vi "SVFA Zoom Power Spectral Density (1 Ch).vi"(0 "scaled signal [EU]":waveform(dbl)={"t0"=timestamp(0 s since 1904-01-01), "dt"=0.0001, "Y"=[]}, 3 "zoom settings":T2={"frequency range"={"start frequency"=1000.0, "stop frequency"=2000.0}, "window"=1, "number of lines"=400, "% overlap"=0.0} {"% overlap" min=0.0 format="%.2f"; "number of lines" min=2; "window" items=["None ", "Hanning", "Hamming", "Blackman-Harris", "Exact Blackman", "Blackman", "Flat Top", "4 Term B-Harris ", "7 Term B-Harris", "Low Sidelobe"]; "frequency range"."stop frequency" min=0.0 format="%.2f"; "frequency range"."start frequency" min=0.0 format="%.2f"}, 4 "dB On (F)":bool, 5 "error in (no error)":errorcluster, 6 "desired units":enum16{"EU^2 / Hz", "EU / sqrt(Hz)"}(ring), 7 "averaging parameters":T1={"averaging mode"=enum."No averaging", "weighting mode"=enum."Exponential", "number of averages"=10, "linear mode"=enum."One shot"} {"number of averages" min=1 step=1}, 9 "restart averaging (F)":bool) -> (11 "averaging done":bool, 12 "new spectrum available":bool, 13 "averages completed":dbl, 14 "power spectral density [EU^2 rms / Hz]":cluster{"f0":dbl, "df":dbl, "magnitude":dbl[]}={"f0"=nan, "df"=inf, "magnitude"=[]} {"magnitude" format="%.2p"; "df" format="%.2p"; "f0" format="%.2p"}, 15 "unit label":string, 18 "spectrum info":T3={"channel name"="", "description"="", "x-axis units"=1, "spectral info"={"spectrum type"=enum."Power [Magnitude^2]", "linear/dB"=enum."linear", "window"=0, "window size"=0, "FFT size"=0}, "engineering units"=0, "custom label"="", "dB reference [EU]"=0.0, "peak units"=enum."rms", "weighting filter"=0, "spectral density?"=FALSE, "unit label"="", "spectrum skewed?"=FALSE, "complimentary spectrum units"=enum."none"} {"x-axis units" items=["Time (s)"=0, "Frequency-CB (Hz)"=1, "Frequency-CPB (Hz)"=1248, "Frequency-Arbitrary (Hz)"=2357, "Quefrency (s)"=2, "Revolutions (rev)"=3, "Order"=4, "Speed (RPM)"=11, "Speed (rad/s)"=21, "Index"=65535]; "weighting filter" items=["Linear", "A-weighting", "B-weighting", "C-weighting", "ITU-R 468-4", "Dolby", "CCITT", "C-message", "Wb", "Wc", "Wd", "We", "Wf", "Wh", "Wj", "Wk", "Wm", "AES17 20 kHz lowpass", "AES17 40 kHz lowpass", "AES17 20 kHz highpass", "AES17 40 kHz highpass"]; "dB reference [EU]" format="%.2f"; "engineering units" items=["custom..."=0, "V"=1, "A"=21, "C"=30, "pC"=31, "s"=32, "-"=29, "Pa"=2, "N"=20, "g"=3, "m/s^2"=4, "m/s"=5, "m"=6, "mm/s"=12, "mm"=13, "micron/s"=14, "micron"=15, "in/s^2"=7, "in/s"=8, "in"=9, "mil/s"=10, "mil"=11, "rad/s^2"=16, "rad/s"=17, "rad"=18, "deg/s^2"=26, "deg/s"=27, "deg"=28, "RPM"=22, "cycle/s^2"=23, "Hz"=24, "cycle"=25, "strain"=19]; "spectral info"."window" items=["None "=0, "Hanning"=1, "Hamming"=2, "Blackman-Harris"=3, "Exact Blackman"=4, "Blackman"=5, "Flat Top"=6, "4 Term B-Harris "=7, "7 Term B-Harris"=8, "Low Sidelobe"=9, "Force - Exponential"=10, "Gaussian"=62]}, 19 "error out":errorcluster)   [LabVIEW 2017]
doc: "Computes the zoom power spectral density of <B>scaled signal [EU]</B> and <B>zoom settings</B>. Data accumulates each time this VI is called. However, it returns a new spectrum only when sufficient data accumulates. Indicators and subsequent processing should only be called when <B>new spectrum available</B> is TRUE. Wire data to the <B>scaled signal [EU]</B> input to determine the polymorphic instance to use or manually select the instance."
uses:
  <vilib>/addons/_NISVFA/_Shared subVIs/Controls/svc_Spectrum Info.ctl
  <vilib>/addons/_NISVFA/_Shared subVIs/Controls/svc_X-Axis Units.ctl
  <vilib>/addons/_NISVFA/_Shared subVIs/Controls/svc_Spectrum Type.ctl
  <vilib>/addons/_NISVFA/_Shared subVIs/Controls/svc_Engineering Units Text Ring.ctl
  <vilib>/addons/_NISVFA/_Shared subVIs/Controls/svc_Weighting Filter Text Ring.ctl
  <vilib>/addons/_NISVFA/_Shared subVIs/Controls/svc_Complimentary Spectrum Units.ctl
  <vilib>/addons/_NISVFA/_Spectrum Processing/SVFA Unit Conversion (1 Ch).vi
  <vilib>/addons/_NISVFA/_Shared subVIs/Common/svc_Get SV Channel Info.vi
  <vilib>/addons/_NISVFA/_Shared subVIs/Common/svc_Spectrum Units.vi
  <vilib>/addons/_NISVFA/_Shared subVIs/Spectrum Averaging/svfa_Reset Averaging State Info.vi
  <vilib>/addons/_NISVFA/_Shared subVIs/Spectrum Averaging/svfa_Average Array with Avg Checks (complex) No State.vi
  <vilib>/addons/_NISVFA/_Shared subVIs/Common/svc_Complex to Mag2 Array.vi
  <vilib>/addons/_NISVFA/_Shared subVIs/Spectrum Averaging/svfa_Average Array with Avg Checks (real) No State.vi
  <vilib>/addons/_NISVFA/_Spectrum Processing/subVIs/svfa_Conversion Utility (spectrum info).vi
  <vilib>/addons/_NISVFA/_Shared subVIs/Spectrum Averaging/svfa_Average Array (complex) No State.vi
  <vilib>/addons/_NISVFA/_Shared subVIs/Spectrum Averaging/svfa_Average Array (real) No State.vi
  <vilib>/addons/_NISVFA/_Spectrum Processing/subVIs/svfa_Peak to RMS to Peak2Peak.vi
  <vilib>/addons/_NISVFA/_Spectrum Processing/subVIs/svfa_Mag to Mag2.vi
  <vilib>/addons/_NISVFA/_Spectrum Processing/subVIs/svfa_Linear to dB.vi
  <vilib>/addons/_NISVFA/_Spectrum Processing/subVIs/svfa_dBrefA to dBrefB.vi
  <vilib>/addons/_NISVFA/_Spectrum Processing/subVIs/svfa_Spectrum to Spectral Density.vi
  <vilib>/addons/_NISVFA/_Shared subVIs/Spectrum Averaging/svfa_No Average Array (complex).vi
  <vilib>/addons/_NISVFA/_Shared subVIs/Spectrum Averaging/svfa_Average Array (complex).vi
  <vilib>/addons/_NISVFA/_Shared subVIs/Spectrum Averaging/svfa_No Average Array (real).vi
  <vilib>/addons/_NISVFA/_Shared subVIs/Spectrum Averaging/svfa_Average Array (real).vi
  <vilib>/addons/_NISVFA/_Shared subVIs/Spectrum Averaging/svfa_Peak Hold Array.vi
  <vilib>/addons/_NISVFA/_Shared subVIs/Common/svc_Get Weighting Enum and Labels.vi
  <vilib>/addons/_NISVFA/_Shared subVIs/Common/svc_Unit Label Lexical Class.vi
  <vilib>/addons/_NISVFA/_Shared subVIs/Common/svc_Engineering Units to Unit Label.vi
  <vilib>/addons/_NISVFA/_Shared subVIs/Common/svc_Format Value (DBL).vi
  <vilib>/addons/_NISVFA/_Shared subVIs/Common/svc_Window Parameters.vi
  <vilib>/addons/_NISVFA/_Shared subVIs/Common/svc_Channel Info to Spectrum Info.vi
  <vilib>/addons/_NISVFA/_Shared subVIs/Common/svc_Unit Label to Engineering Units.vi
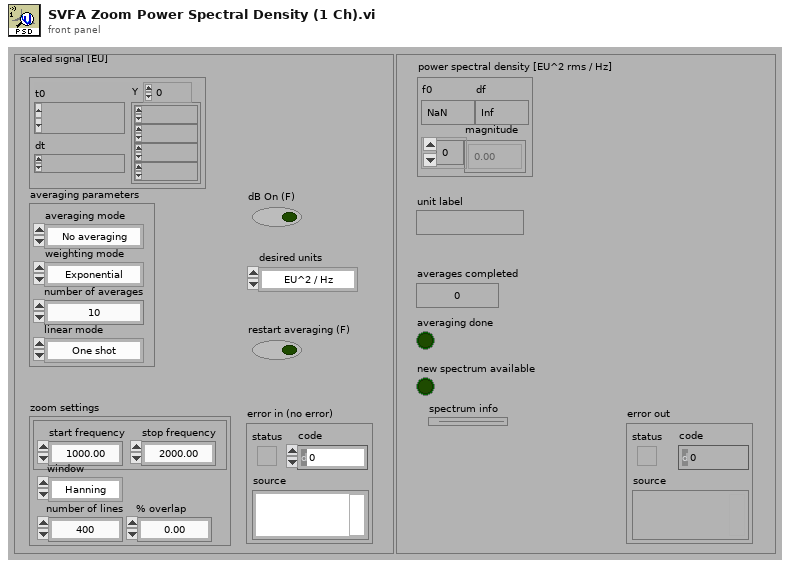
[diagram p1: front panel]
types:
  T1 = cluster{"averaging mode":enum16{"No averaging", "Vector averaging", "RMS averaging", "Peak hold"}, "weighting mode":enum16{"Linear", "Exponential"}, "number of averages":u32, "linear mode":enum16{"One shot", "Auto restart"}}
  T2 = cluster{"frequency range":cluster{"start frequency":dbl, "stop frequency":dbl}, "window":u16, "number of lines":i32, "% overlap":dbl}
  T3 = typedef "svc_Spectrum Info.ctl" = cluster{"channel name":string, "description":string, "x-axis units":T4, "spectral info":cluster{"spectrum type":T5, "linear/dB":enum16{"linear", "dB"}, "window":u16, "window size":i32, "FFT size":i32}, "engineering units":T6, "custom label":string, "dB reference [EU]":dbl, "peak units":enum16{"rms", "peak", "peak-peak"}, "weighting filter":T7, "spectral density?":bool, "unit label":string, "spectrum skewed?":bool, "complimentary spectrum units":T8}
  T4 = typedef "svc_X-Axis Units.ctl" = u16
  T5 = typedef "svc_Spectrum Type.ctl" = enum16{"FFT Spectrum [complex]", "Amplitude [Magnitude]", "Power [Magnitude^2]", "Cross Spectrum [complex]", "Frequency Response [Complex]"}
  T6 = typedef "svc_Engineering Units Text Ring.ctl" = u16
  T7 = typedef "svc_Weighting Filter Text Ring.ctl" = u16
  T8 = typedef "svc_Complimentary Spectrum Units.ctl" = enum16{"none", "radians", "degrees", "cycles", "imaginary"}
  T9 = enum16{"Restart processing", "Continue processing", "Skip processing"}
  T10 = enum16{"No averaging", "Vector averaging", "RMS averaging", "Peak hold"}
  T11 = cluster{"linear/dB":enum16{"no change", "linear", "dB"}, "dB reference (0: no change)":dbl, "power/magnitude":enum16{"no change", "power", "magnitude"}, "view":enum16{"no change", "rms", "peak", "peak-peak"}}
  T12 = enum16{"no change", "spectrum", "spectral density"}
  T13 = cluster{"zoom settings":cluster{"center frequency":dbl, "zoom":i32, "trim":dbl}, "FFT settings":cluster{"window":enum16{"None ", "Hanning", "Hamming", "Blackman-Harris", "Exact Blackman", "Blackman", "Flat Top", "4 Term B-Harris ", "7 Term B-Harris", "Low Sidelobe"}, "window size":i32, "FFT size":i32, "%overlap":dbl}}
  T14 = cluster{"complex FFT":cdb[], "real FFT":dbl[], "f0":dbl, "df":dbl, "averages completed":dbl, "averaging parameters":cluster{"averaging mode":enum16{"No averaging", "Vector averaging", "RMS averaging", "Peak hold"}, "weighting mode":enum16{"Linear", "Exponential"}, "number of averages":u32, "linear mode":enum16{"One shot", "Auto restart"}}}
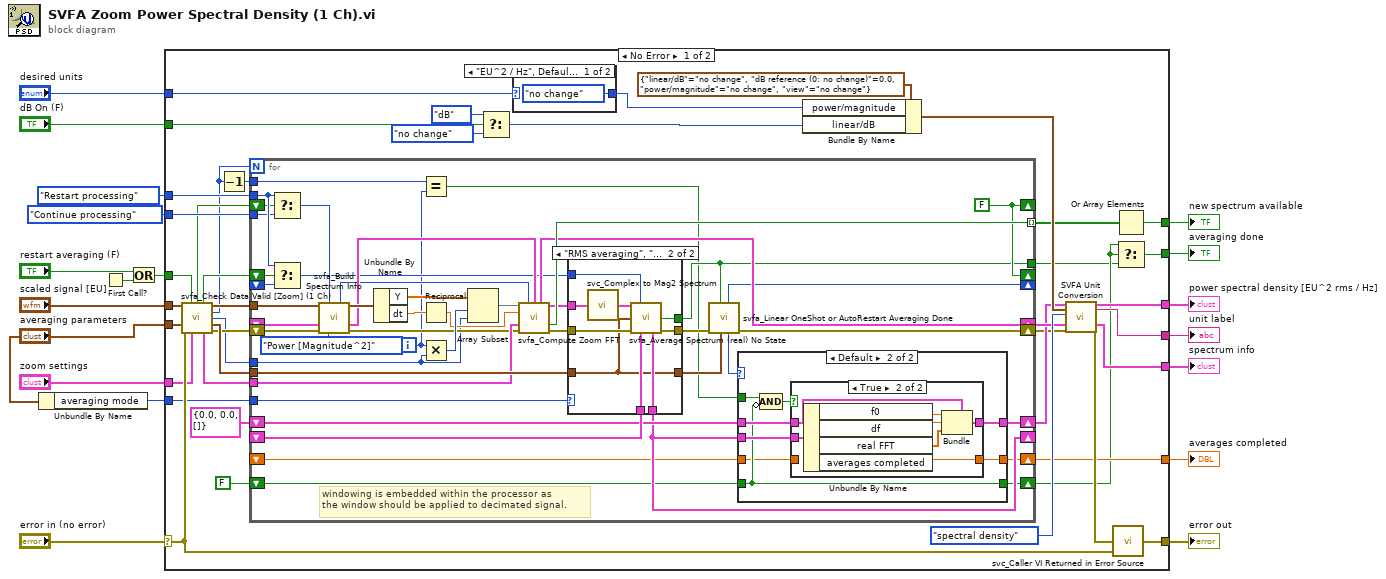
[diagram p0: block diagram]
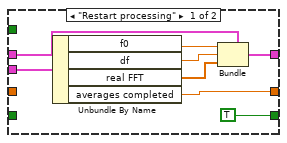
[diagram p2: hidden frame]
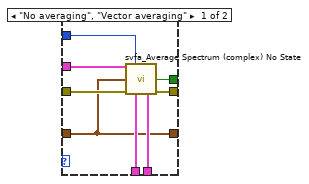
[diagram p4: hidden frame]
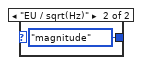
[diagram p5: hidden frame]
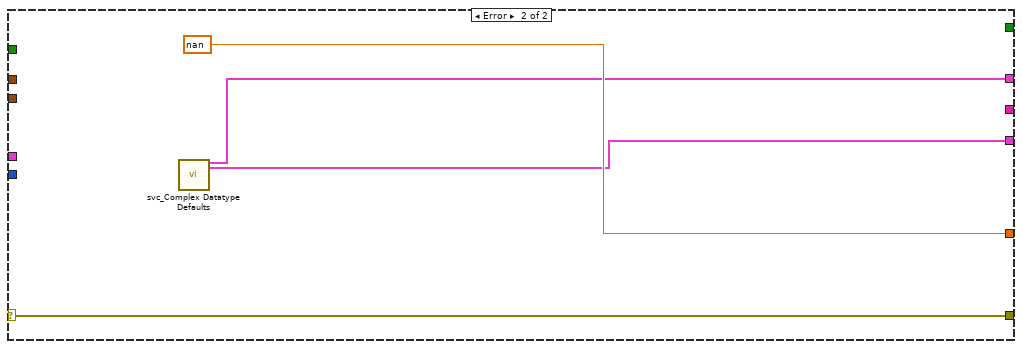
[diagram p6: hidden frame]
diagram:
  n1 = Unbundle By Name("averaging parameters") -> ("averaging mode"=w1:T10)
  n2 = First Call?() -> (First Call?: T/F=w8:bool)
  n3 = Or(x="restart averaging (F)", y=w8) -> (x .or. y?=w6:bool)
  n4 = case shown="No Error" "error in (no error)" {
    tunnel: [w24 nan ("Averaged So-far")] -> w18
    tunnel: [w60 w152] -> w14
    tunnel: "averaging parameters" -> [w56 _]
    tunnel: "zoom settings" -> [w41 _]
    tunnel: "scaled signal [EU]" -> [w61 _]
    tunnel: [w58 _] -> w13
    tunnel: "dB On (F)" -> [w47 _]
    tunnel: [w57 w151] -> w12
    tunnel: w6 -> [w34 _]
    tunnel: "desired units" -> [w48 _]
    selector: "error in (no error)" -> [w54 w154]
    tunnel: [w55 w154] -> w16
    tunnel: [w35 _] -> w17
    tunnel: [w22 _] -> w10
    tunnel: T9."Restart processing" ("processing control") -> [w33 _]
    tunnel: T9."Continue processing" ("processing control") -> [w32 _]
    tunnel: w1 -> [w30 _]
    frame No Error {
      n5 = call <vilib>:"svfa_Check Data Valid [Zoom] (1 Ch).vi"("signal [V]"=w61, "restart averaging (F)"=w34, "averaging parameters"=w56, "error in (no error)"=w54, "zoom settings"=w41) -> ("reset processing"=w31:bool, "restart averaging"=w39:bool, "dup signal [V]"=w44:waveform(dbl), "iterations"=w29:i32, "maximum block size"=w36:i32, "dup averaging parameters"=w43:T1, "zoom FFT settings"=w40:T13, "error out"=w42:errorcluster)  [unwired: 3 in]
      n6 = Decrement(x=w29) -> (x-1=w28:i32)
      n7 = for {
        N: w29 -> [_]
        tunnel: [w105] -> w38 mode=indexing
        tunnel: w44 -> [w106]
        tunnel: [w74] -> w21
        shift-left: _ -> [w102]
        shift-right: [w70] -> _
        shift-right: [w104] -> w37
        shift-left: _ -> [w103]
        tunnel: w43 -> [w101]
        shift-right: [w73] -> _
        shift-left: _ -> [w99]
        tunnel: w33 -> [w95]
        tunnel: w40 -> [w97]
        shift-right: [w76] -> _
        shift-left: w39 -> [w98]
        tunnel: w36 -> [w75]
        tunnel: w32 -> [w94]
        shift-right: [w76] -> _
        shift-left: w31 -> [w93]
        tunnel: w30 -> [w78]
        shift-right: [w72] -> w25
        shift-left: cluster{"f0":dbl, "df":dbl, "real FFT":dbl[]} {"f0"=0.0, "df"=0.0, "real FFT"=[]} -> [w71]
        tunnel: w28 -> [w69]
        shift-right: [w65] -> w24
        shift-left: _ -> [w64]
        shift-right: [w66] -> w23
        shift-left: FALSE ("restart averaging") -> [w63]
        shift-right: [w62] -> w20
        shift-left: w42 -> [w100]
        i -> [w68]
        w76 = FALSE ("restart averaging")
        # "windowing is embedded within the processor as \nthe window should be applied to decimated signal."
        n8 = Select(t=w95, s=w93, f=w94) -> (s? t:f=w80:T9)
        n9 = Select(t=w95, s=w98, f=w99) -> (s? t:f=w79:T9)
        n10 = call <vilib>:"svfa_Build Spectrum Info.vi"("scaled signal [EU]"=w106, "processing control"=w80, "spectrum info in"=w103, "error in (no error)"=w100, "spectrum type"=svc_Spectrum_Type."Power [Magnitude^2]") -> ("dup processing control"=w85:T9, "dup scaled signal [EU]"=w91:waveform(dbl), "spectrum info out"=w89:T3, "error out"=w83:errorcluster)  [unwired: 7 in]
        n11 = Unbundle By Name ("Get Waveform Components")(w91) -> ("Y"=w82:dbl[], "dt"=w90:dbl)
        n12 = Equal?(x=w69, y=w68) -> (x = y?=w67:bool)
        n13 = Reciprocal(x=w90) -> (1/x=w84:dbl)
        n14 = Multiply(x=w68, y=w75) -> (x*y=w96:i32)
        n15 = Array Subset(array=w82, index=w96, length=w75) -> (w81:dbl[])
        n16 = call <vilib>:"svfa_Compute Zoom FFT.vi"("x"=w81, "processing control"=w85, "spectrum info"=w89, "fs"=w84, "zoom FFT settings"=w97, "error in (no error)"=w83) -> ("spectrum info out"=w104:T3, "FFT spectrum"=w88:cluster{"f0":dbl, "df":dbl, "spectrum":cdb[]}, "spectrum ready"=w105:bool, "error out"=w87:errorcluster)  [unwired: 5 in, 1 out]
        n17 = case shown="\"RMS averaging\", \"Peak hold\"" w78 {
          tunnel: w101 -> [w132 w140]
          tunnel: [w137 w146] -> w92
          tunnel: [w136 w147] -> w74
          tunnel: w88 -> [w139 w145]
          tunnel: w87 -> [w138 w148]
          tunnel: w79 -> [w135 w143]
          tunnel: w102 -> [w134 w141]
          tunnel: [w133 w142] -> w70
          tunnel: [w132 w140] -> w77
          frame "No averaging", "Vector averaging" {
            n18 = call <vilib>:"svfa_Average Spectrum (complex) No State.vi"("spectrum"=w139, "processing control"=w135, "averaging parameters"=w132, "error in (no error)"=w138, "averaging state info in"=w134) -> ("averaging done"=w136:bool, "averaging state info out"=w133:T14, "error out"=w137:errorcluster)  [unwired: 5 in, 3 out]
          }
          frame "RMS averaging", "Peak hold" {
            n19 = call <vilib>:"svc_Complex to Mag2 Spectrum.vi"("complex spectrum"=w145) -> ("power spectrum"=w144:cluster{"f0":dbl, "df":dbl, "spectrum":dbl[]})  [unwired: 4 in]
            n20 = call <vilib>:"svfa_Average Spectrum (real) No State.vi"("spectrum"=w144, "processing control"=w143, "averaging parameters"=w140, "error in (no error)"=w148, "averaging state info in"=w141) -> ("averaging done"=w147:bool, "averaging state info out"=w142:T14, "error out"=w146:errorcluster)  [unwired: 5 in, 3 out]
          }
        }
        n21 = call <vilib>:"svfa_Linear OneShot or AutoRestart Averaging Done.vi"("averaging parameters"=w77, "averaging done"=w74, "error in (no error)"=w92) -> ("error out"=w62:errorcluster, "processing control"=w73:T9)  [unwired: 7 in]
        n22 = case shown="Default" w73 {
          tunnel: w70 -> [w111 w122]
          tunnel: [TRUE ("restart averaging") w117] -> w66
          tunnel: [w109 w121] -> w72
          tunnel: w63 -> [_ w117]
          tunnel: w67 -> [_ w120]
          tunnel: w71 -> [w108 w119]
          tunnel: [w107 w116] -> w65
          tunnel: w64 -> [_ w115]
          frame "Restart processing" {
            n23 = Unbundle By Name(w111) -> ("f0"=w114:dbl, "df"=w113:dbl, "real FFT"=w112:dbl[], "averages completed"=w107:dbl)
            n24 = Bundle(cluster=w108, "f0"=w114, "df"=w113, "real FFT"=w112) -> (w109:cluster{"f0":dbl, "df":dbl, "real FFT":dbl[]})
          }
          frame Default {
            n25 = Compound Arithmetic op=AND(w120, invert w117) -> (w118:bool)
            n26 = case shown="True" w118 {
              tunnel: w122 -> [_ w128]
              tunnel: [w124 w127] -> w121
              tunnel: w119 -> [w124 w126]
              tunnel: [w123 w125] -> w116
              tunnel: w115 -> [w123 _]
              frame False {
              }
              frame True {
                n27 = Unbundle By Name(w128) -> ("f0"=w131:dbl, "df"=w130:dbl, "real FFT"=w129:dbl[], "averages completed"=w125:dbl)
                n28 = Bundle(cluster=w126, "f0"=w131, "df"=w130, "real FFT"=w129) -> (w127:cluster{"f0":dbl, "df":dbl, "real FFT":dbl[]})
              }
            }
          }
        }
      }
      n29 = Select(t=enum16{"no change", "linear", "dB"}."dB" ("linear/dB"), s=w47, f=enum16{"no change", "linear", "dB"}."no change" ("linear/dB")) -> (s? t:f=w51:enum16{"no change", "linear", "dB"})
      n30 = case shown="\"EU^2 / Hz\", Default" w48 {
        tunnel: [enum16{"no change", "power", "magnitude"}."no change" ("power/magnitude") enum16{"no change", "power", "magnitude"}."magnitude" ("power/magnitude")] -> w53
        frame "EU^2 / Hz", Default {
        }
        frame "EU / sqrt(Hz)" {
        }
      }
      n31 = Bundle By Name(cluster=T11 {"linear/dB"=enum."no change", "dB reference (0: no change)"=0.0, "power/magnitude"=enum."no change", "view"=enum."no change"} ("desired scaling"), "power/magnitude"=w53, "linear/dB"=w51) -> (w46:T11)
      n32 = call-poly <vilib>:"SVFA Unit Conversion.vi"("spectrum"=w25, "desired scaling"=w46, "spectral density desired"=T12."spectral density", "spectrum info in"=w37, "error in (no error)"=w20) -> ("converted spectrum"=w60:cluster{"x0":dbl, "dx":dbl, "magnitude":dbl[]}, "unit label"=w58:string, "spectrum info out"=w57:T3, "error out"=w59:errorcluster)  [unwired: 11 in]
      n33 = call <vilib>:"svc_Caller VI Returned in Error Source.vi"("warning input to caller"=w54, "error in (no error)"=w59) -> ("error out"=w55:errorcluster)  [unwired: 3 in]
      n34 = Or Array Elements(Boolean array=w38) -> (logical OR=w35:bool)
      n35 = Select(t=w23, s=w23, f=w21) -> (s? t:f=w22:bool)
    }
    frame Error {
      n36 = call <vilib>:"svc_Complex Datatype Defaults.vi"() -> ("empty spectrum"=w152:cluster{"f0":dbl, "df":dbl, "magnitude":dbl[]}, "dead spectrum info"=w151:T3)  [unwired: 11 in, 7 out]
    }
  }
  "averages completed" <- w18
  "new spectrum available" <- w17
  "error out" <- w16
  "power spectral density [EU^2 rms / Hz]" <- w14
  "unit label" <- w13
  "spectrum info" <- w12
  "averaging done" <- w10
